vi "Keithley6221 Ramp DC Current.vi"(6 "stop":bool, 7 "Sweep Time (H:M:S)":dbl=3600.0 format="%<%H:%M:%S>t", 8 "Mapping":bool, 9 "End Current (A)":dbl=1e-10 format="%.3e", 10 "Start Current (A)":dbl=1e-06 format="%.3e", 11 "K6221 GPIB address":refnum<visa-resource-name>) -> (4 "Last Sent Value":dbl=1e-06 format="%.3e")   [LabVIEW 2024]
uses:
  Global Variables/Current K6221 Coarse.vi
panel:
  in  "Time interval (sec)":dbl=0.5 min=0.1 step=0.1
  out "Numeric":i32
  out "Prepared Value":dbl=1e-06 format="%.3e"
  # "Log"
  # "Linear"
  # "Add two extra sec for timing."
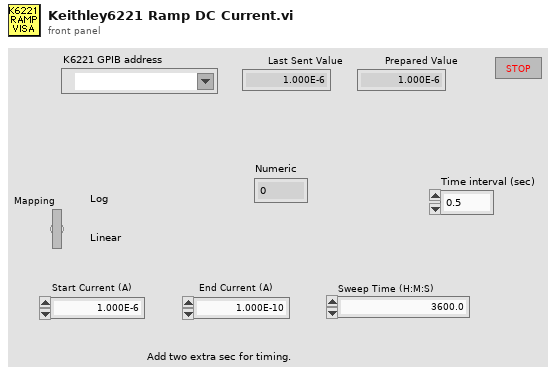
[diagram p1: front panel]
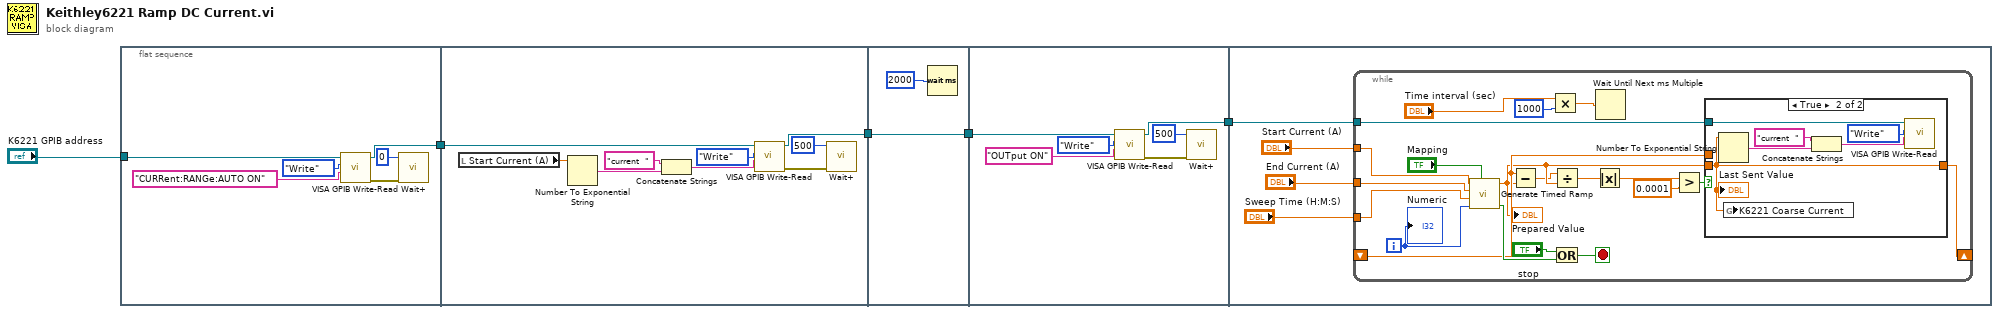
[diagram p0: block diagram]
diagram:
  n1 = flat-sequence {
    tunnel: "K6221 GPIB address" -> [w7]
    tunnel: [w6] -> w4
    tunnel: w4 -> [w13]
    tunnel: [w12] -> w3
    tunnel: w3 -> [w21]
    tunnel: [w21] -> w2
    tunnel: w2 -> [w24]
    tunnel: [w23] -> w1
    tunnel: w1 -> [w30]
    frame #0 {
      n2 = call "VISA GPIB Write-Read.vi"("Command"="CURRent:RANGe:AUTO ON" ("String to Write"), "Action"=enum16{"Write", "Read", "Write & Read"}."Write", "VISA resource name"=w7) -> ("error out"=w8:errorcluster, "dup VISA Session"=w6:refnum<visa-resource-name>)  [unwired: 5 in, 2 out]
      n3 = call "Wait+.vi"("Error In"=w8, "milliseconds to wait"=u32 0) -> ()  [unwired: 4 in, 2 out]
    }
    frame #1 {
      n4 = local read "Start Current (A)"() -> (w16:dbl)
      n5 = Number To Exponential String(number=w16) -> (E-format string=w18:string)  [unwired: 3 in]
      n6 = Concatenate Strings("current  " ("initial string"), w18) -> (w17:string)
      n7 = call "VISA GPIB Write-Read.vi"("Command"=w17, "Action"=enum16{"Write", "Read", "Write & Read"}."Write", "VISA resource name"=w13) -> ("error out"=w14:errorcluster, "dup VISA Session"=w12:refnum<visa-resource-name>)  [unwired: 5 in, 2 out]
      n8 = call "Wait+.vi"("Error In"=w14, "milliseconds to wait"=u32 500) -> ()  [unwired: 4 in, 2 out]
    }
    frame #2 {
      n9 = Wait (ms)(milliseconds to wait=u32 2000) -> ()  [unwired: 1 out]
    }
    frame #3 {
      n10 = call "VISA GPIB Write-Read.vi"("Command"="OUTput ON" ("String to Write"), "Action"=enum16{"Write", "Read", "Write & Read"}."Write", "VISA resource name"=w24) -> ("error out"=w25:errorcluster, "dup VISA Session"=w23:refnum<visa-resource-name>)  [unwired: 5 in, 2 out]
      n11 = call "Wait+.vi"("Error In"=w25, "milliseconds to wait"=u32 500) -> ()  [unwired: 4 in, 2 out]
    }
    frame #4 {
      n12 = while {
        tunnel: "Start Current (A)" -> [w52]
        tunnel: "End Current (A)" -> [w51]
        tunnel: "Sweep Time (H:M:S)" -> [w50]
        shift-right: [w43] -> _
        shift-left: _ -> [w41]
        tunnel: w30 -> [w39]
        i -> [w49]
        stop <- w47 stop-if-true
        n13 = call "Generate Timed Ramp.vi"("Log"="Mapping", "Point #"=w49, "Time (Hr:Min:Sec)"=w50, "Stop"=w51, "Start"=w52) -> ("Stop"=w46:bool, "Output"=w40:dbl)  [unwired: 2 out]
        "Prepared Value" <- w40
        n14 = Subtract(x=w41, y=w40) -> (x-y=w33:dbl)
        n15 = Multiply(x="Time interval (sec)", y=u32 1000 ("millisecond multiple")) -> (x*y=w37:dbl)
        n16 = Divide(x=w33, y=w40) -> (x/y=w35:dbl)
        n17 = Or(x="stop", y=w46) -> (x .or. y?=w47:bool)
        n18 = Absolute Value(x=w35) -> (abs(x)=w34:dbl)
        n19 = Wait Until Next ms Multiple(millisecond multiple=w37) -> ()  [unwired: 1 out]
        n20 = Greater?(x=w34, y=0.0001) -> (0:w42:bool)
        n21 = case shown="True" w42 {
          tunnel: [w53 w54] -> w43
          tunnel: w41 -> [w53 _]
          tunnel: w40 -> [_ w54]
          tunnel: w39 -> [_ w58]
          frame False {
          }
          frame True {
            n22 = Number To Exponential String(number=w54) -> (E-format string=w55:string)  [unwired: 3 in]
            n23 = global write "Current K6221 Coarse.vi" "K6221 Coarse Current"(w54) -> ()
            n24 = Concatenate Strings("current  " ("initial string"), w55) -> (w57:string)
            n25 = call "VISA GPIB Write-Read.vi"("Command"=w57, "Action"=enum16{"Write", "Read", "Write & Read"}."Write", "VISA resource name"=w58) -> ()  [unwired: 5 in, 4 out]
            "Last Sent Value" <- w54
          }
        }
        "Numeric" <- w49
      }
    }
  }
